vi "Create Default Input.vi"(3 "Input":refnum<class "Input.lvclass">, 11 "Default Value":variant) -> ()   [LabVIEW 2020, in "Parallel Block.lvlib" / "Manager.lvclass"]
uses:
  Manager.lvclass
  Manager.lvclass/Manager.ctl
  Input/Input.lvclass
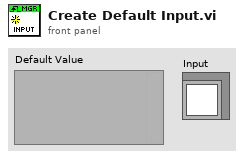
[diagram p1: front panel]
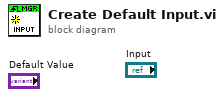
[diagram p0: block diagram]
diagram:
